vi "Parse Layout-VI for SubPanels.vi"(8 "error in (no error)":errorcluster, 11 "Layout-VI Ref":refnum<vi>) -> (0 "error out":errorcluster, 3 "SubPanels":T1)   [LabVIEW 2022 SP3, in "UI Manager.lvlib"]
doc: "Parse the Layout VI <b>in</b> and identify all the SubPanels within it and produce a SubPanel Map <b>out</b> with the SubPanel names as the Keys, and SubPanel references and blank VI refernces as attributes.\n\n____\nHAMPEL SOFTWARE ENGINEERING v2.6.0 (2023-12-19 10:54)"
uses:
  UI Manager.lvlib
  SubPanels--map.ctl
  SubPnl Map References--cluster.ctl
  <vilib>/Hampel Software Engineering/HSE Logger/hse-logger.lvlib
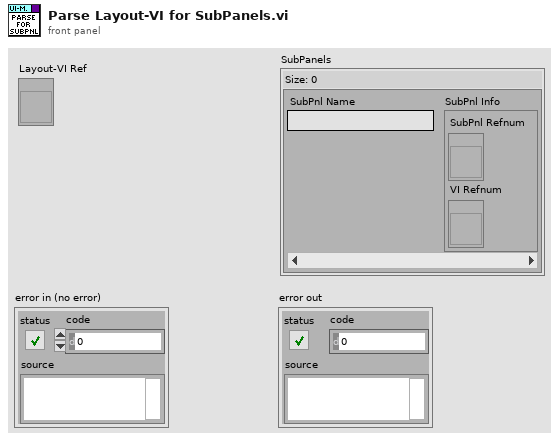
[diagram p1: front panel]
types:
  T1 = typedef "UI Manager.lvlib/SubPanels--map.ctl" = map{string, T2}
  T2 = typedef "UI Manager.lvlib/SubPnl Map References--cluster.ctl" = cluster{"SubPnl Refnum":refnum<vi>, "VI Refnum":refnum<vi>}
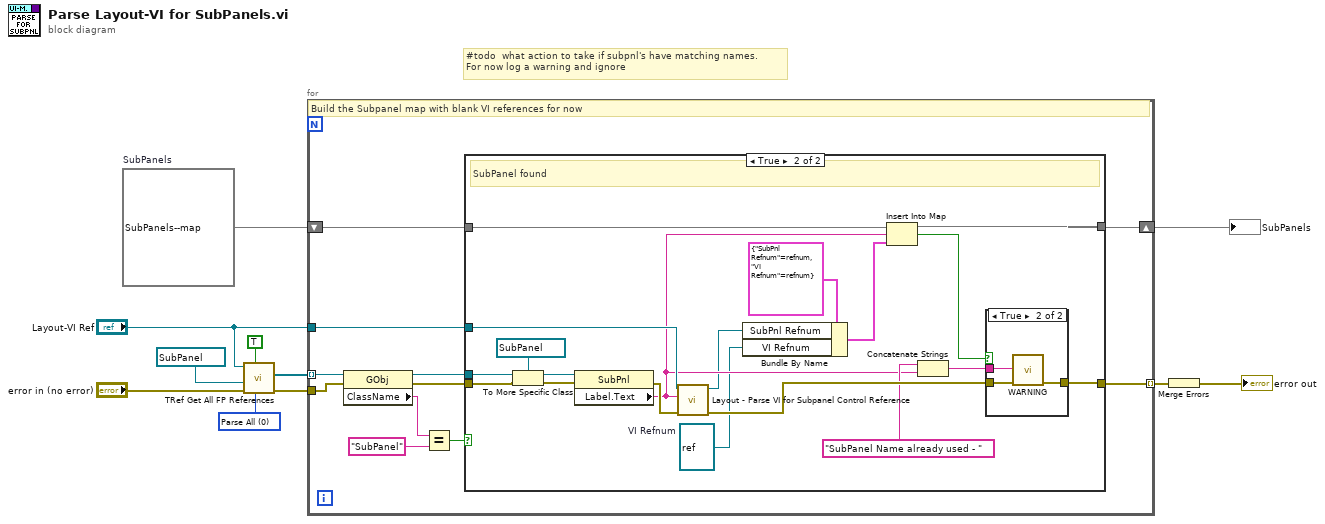
[diagram p0: block diagram]
diagram:
  w11 = u16 0 items=["Parse All", "Parse Tabs Only"] ("Parsing Rule")
  w5 = T1 {}  # SubPanels
  # "#todo  what action to take if subpnl's have matching names.\nFor now log a warning and ignore"
  n1 = call <vilib>:"TRef Get All FP References.vi"("Parsing Rule"=w11, "Ignore Decorations?"=TRUE, "error in (no error)"="error in (no error)", "GObj Refnum"=refnum<vi> refnum ("SubPnl Refnum"), "VI Refnum"="Layout-VI Ref") -> ("error out"=w7:errorcluster, "All FP Objects"=w6:refnum<vi>[])  [unwired: 2 in, 3 out]
  n2 = for {
    tunnel: w7 -> [w21]
    tunnel: w6 -> [w22] mode=indexing
    tunnel: "Layout-VI Ref" -> [w15]
    shift-right: [w13] -> w3
    shift-left: w5 -> [w14]
    tunnel: [w12] -> w2 mode=indexing
    # "Build the Subpanel map with blank VI references for now"
    n3 = property class="GObj"(reference=w22, error in=w21) -> (reference out=w17:refnum<vi>, error out=w16:errorcluster, "ClassName"=w20:string)
    n4 = Equal?(x=w20, y="SubPanel") -> (x = y?=w18:bool)
    n5 = case shown="True" w18 {
      tunnel: w17 -> [_ w43]
      tunnel: w16 -> [w23 w42]
      tunnel: w15 -> [_ w38]
      tunnel: w14 -> [w24 w37]
      tunnel: [w24 w36] -> w13
      tunnel: [w23 w33] -> w12
      frame False {
      }
      frame True {
        w25 = refnum<vi> refnum  # VI Refnum
        # "SubPanel found"
        n6 = To More Specific Class(target class=refnum<vi> refnum ("SubPnl Refnum"), reference=w43, error in=w42) -> (specific class reference=w41:refnum<vi>, error out=w39:errorcluster)
        n7 = property class="SubPnl"(reference=w41, error in=w39) -> (error out=w32:errorcluster, "Label.Text"=w30:string)  [unwired: 1 out]
        n8 = call "Layout - Parse VI for Subpanel Control Reference.vi"("error in (no error)"=w32, "SubPanel Label"=w30, "VI in"=w38) -> ("error out"=w34:errorcluster, "SubPanel Ref"=w26:refnum<vi>)  [unwired: 7 in]
        n9 = Bundle By Name(cluster=T2 {"SubPnl Refnum"=refnum, "VI Refnum"=refnum} ("value"), "SubPnl Refnum"=w26, "VI Refnum"=w25) -> (w27:T2)
        n10 = Insert Into Map(map in=w37, key=w30, value=w27) -> (map out=w36:T1, key already included?=w35:bool)  [unwired: 1 out]
        n11 = Concatenate Strings("SubPanel Name already used - ", w30) -> (w29:string)
        n12 = case shown="True" w35 {
          tunnel: w34 -> [w44 w47]
          tunnel: [w44 w46] -> w33
          tunnel: w29 -> [_ w45]
          frame False {
          }
          frame True {
            n13 = call <vilib>:"WARNING.vi"("Message"=w45, "error in"=w47) -> ("error out"=w46:errorcluster)  [unwired: 9 in]
          }
        }
      }
    }
  }
  "SubPanels" <- w3
  n14 = Merge Errors(w2) -> (→"error out":errorcluster)
